vi "Handle verified serial UI.vi"(9 "serial status":bool, 10 "DataMatrix Text":string, 11 "REF in":T1) -> (3 "REF out":T1)   [LabVIEW 2024]
uses:
  CTRLS/REF.ctl
  CTRLS/Main Tabs.ctl
  CTRLS/Open Batch Data.ctl
  CTRLS/DM_Data.ctl
  CTRLS/run statistics.ctl
  CTRLS/System settings.ctl
  CTRLS/Printer Message settings.ctl
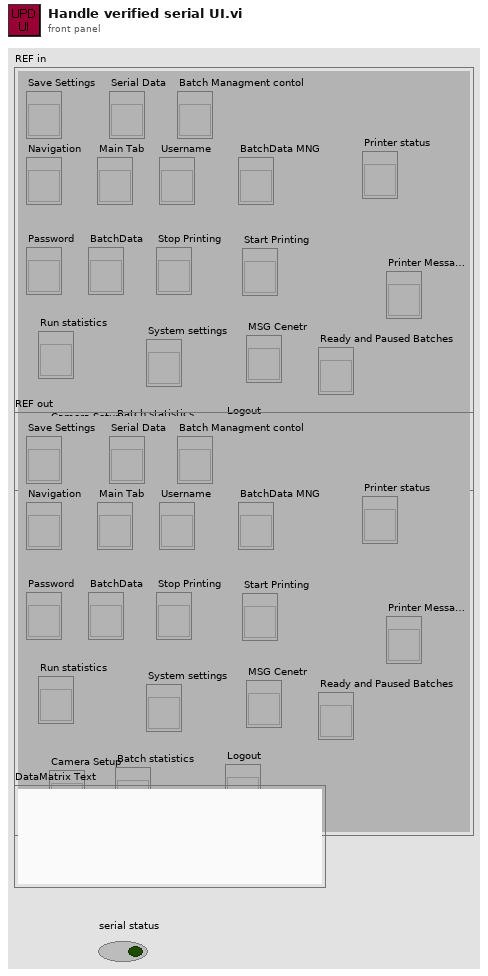
[diagram p1: front panel]
types:
  T1 = typedef "REF.ctl" = cluster{"Save Settings":refnum<vi>, "Navigation":refnum<vi>, "Main Tab":refnum<vi>, "Password":refnum<vi>, "BatchData":refnum<vi>, "Serial Data":refnum<vi>, "Username":refnum<vi>, "Stop Printing":refnum<vi>, "Run statistics":refnum<vi>, "System settings":refnum<vi>, "Batch Managment contol":refnum<vi>, "Start Printing":refnum<vi>, "BatchData MNG":refnum<vi>, "MSG Cenetr":refnum<vi>, "Printer status":refnum<vi>, "Printer Message Config":refnum<vi>, "Ready and Paused Batches":refnum<vi>, "Camera Setup":refnum<vi>, "Batch statistics":refnum<vi>, "Logout":refnum<vi>}
  T2 = typedef "Open Batch Data.ctl" = cluster{"Batch Name":string, "Batch Number":string, "GTIN":string, "Expiry Date":string, "MFG Date":string}
  T3 = cluster{"DM Text":string, "GTIN":string, "Batch":string, "Expiry Date":string, "MFG Date":string, "Serial Number":string, "SSCC":string}
  T4 = typedef "run statistics.ctl" = cluster{"Good":dbl, "Bad":dbl, "Good %":dbl, "Bad %":dbl}
  T5 = typedef "DM_Data.ctl" = cluster{"2D Code String":string, "Batch Number":string, "GTIN":string, "EXP":string, "Serial":string, "MFG":string}
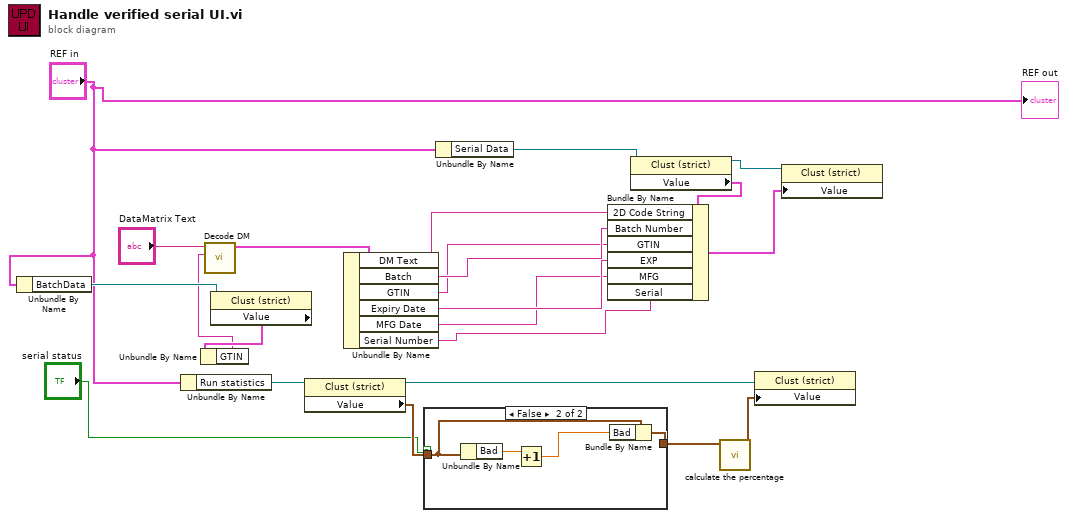
[diagram p0: block diagram]
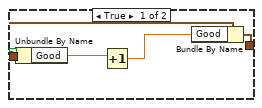
[diagram p2: hidden frame]
diagram:
  n1 = Unbundle By Name("REF in") -> ("BatchData"=w4:refnum<vi>)
  n2 = Unbundle By Name("REF in") -> ("Run statistics"=w10:refnum<vi>)
  n3 = property class="Clust (strict)"(reference=w4) -> ("Value"=w2:T2)  [unwired: 1 in, 2 out]
  n4 = Unbundle By Name(w2) -> ("GTIN"=w1:string)
  n5 = call "Decode DM.vi"("GTIN"=w1, "DataMatrix Text"="DataMatrix Text") -> ("DM CONTENT OUT"=w22:T3)  [unwired: 9 in]
  n6 = property class="Clust (strict)"(reference=w10) -> (reference out=w9:refnum<vi>, "Value"=w8:T4)  [unwired: 1 in, 1 out]
  n7 = Unbundle By Name(w22) -> ("DM Text"=w18:string, "Batch"=w17:string, "GTIN"=w16:string, "Expiry Date"=w15:string, "MFG Date"=w14:string, "Serial Number"=w13:string)
  n8 = case shown="False" "serial status" {
    tunnel: w8 -> [w25 w29]
    tunnel: [w23 w27] -> w7
    frame True {
      n9 = Unbundle By Name(w25) -> ("Good"=w26:dbl)
      n10 = Increment(x=w26) -> (x+1=w24:dbl)
      n11 = Bundle By Name(cluster=w25, "Good"=w24) -> (w23:T4)
    }
    frame False {
      n12 = Unbundle By Name(w29) -> ("Bad"=w30:dbl)
      n13 = Increment(x=w30) -> (x+1=w28:dbl)
      n14 = Bundle By Name(cluster=w29, "Bad"=w28) -> (w27:T4)
    }
  }
  n15 = Unbundle By Name("REF in") -> ("Serial Data"=w21:refnum<vi>)
  n16 = property class="Clust (strict)"(reference=w21) -> (reference out=w12:refnum<vi>, "Value"=w20:T5)  [unwired: 1 in, 1 out]
  n17 = Bundle By Name(cluster=w20, "2D Code String"=w18, "Batch Number"=w17, "GTIN"=w16, "EXP"=w15, "MFG"=w14, "Serial"=w13) -> (w11:T5)
  n18 = call "calculate the percentage.vi"("run statistics in"=w7) -> ("run statistics out"=w6:T4)  [unwired: 10 in]
  n19 = property class="Clust (strict)"(reference=w9, "Value"=w6) -> ()  [unwired: 1 in, 2 out]
  n20 = property class="Clust (strict)"(reference=w12, "Value"=w11) -> ()  [unwired: 1 in, 2 out]
  "REF out" <- "REF in"
